vi "CRYAPI MANAGER.vi"(6 "cSpliterPos":T2(array[cluster]), 8 "tFrame":T3, 9 "sData":string, 10 "nData":i32, 11 "sAction":string) -> (1 "nData_Out":i32, 3 "tFrame_Out":T3)   [LabVIEW 2013]
uses:
  <vilib>/Utility/miscctls.llb/LVRectTypeDef.ctl
  CRYMain Sub Window Global.vi
panel:
  in  "nDocID":i32
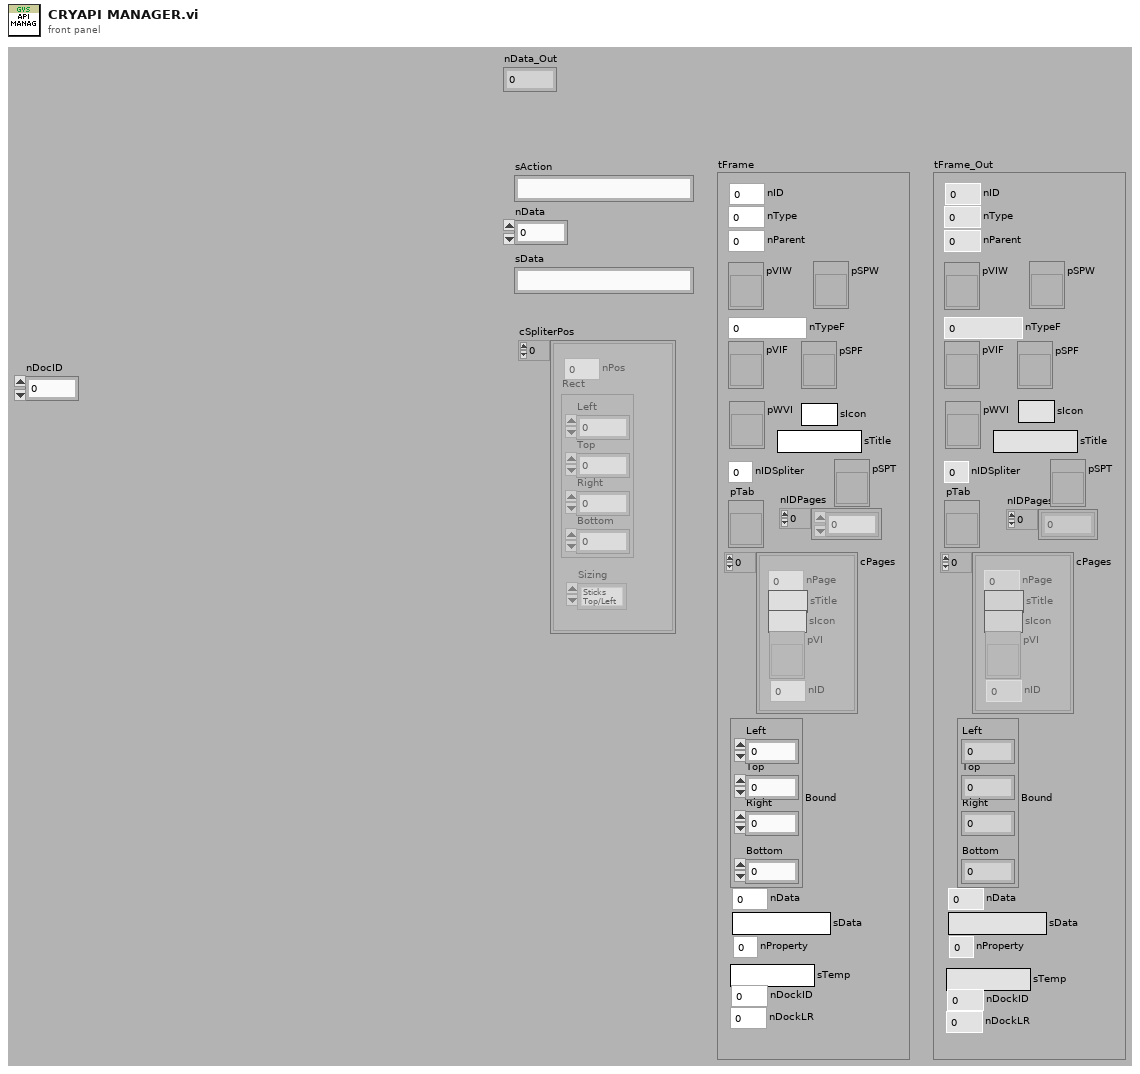
[diagram p1: front panel]
types:
  T1 = typedef "LVRectTypeDef.ctl" = cluster{"Left":i16, "Top":i16, "Right":i16, "Bottom":i16}
  T2 = cluster{"nPos":i32, "Rect":T1, "Sizing":enum16{"Sticks Top/Left", "Sticks Bottom/Right", "Proportional"}}[]
  T3 = cluster{"nType":i32, "nParent":i32, "pVIW":refnum<vi>, "pSPW":refnum<vi>, "nTypeF":i32, "pVIF":refnum<vi>, "pSPF":refnum<vi>, "nIDSpliter":i32, "nProperty":i32, "Bound":T1, "nID":i32, "nData":i32, "sData":string, "pWVI":refnum<vi>, "sTitle":string, "cPages":cluster{"nPage":i32, "sTitle":string, "sIcon":string, "pVI":refnum<vi>, "nID":i32}[], "pTab":refnum<vi>, "nIDPages":i32[], "pSPT":refnum<vi>, "sTemp":string, "nDockID":i32, "nDockLR":i32, "sIcon":string}
  T4 = enum16{"Sticks Top/Left", "Sticks Bottom/Right", "Proportional"}
  T5 = enum32{"Invalid", "Standard", "Closed", "Hidden", "Minimized", "Maximized"}
  T6 = enum32{"Invalid", "Default", "Floating", "Floating/Auto-Hide", "Modal"}
  T7 = cluster{"nPage":i32, "sTitle":string, "sIcon":string, "pVI":refnum<vi>, "nID":i32}[]
  T8 = cluster{"nID":i32[], "Frame":cluster{"nType":i32, "nParent":i32, "pVIW":refnum<vi>, "pSPW":refnum<vi>, "nTypeF":i32, "pVIF":refnum<vi>, "pSPF":refnum<vi>, "nIDSpliter":i32, "nProperty":i32, "Bound":T1, "nID":i32, "nData":i32, "sData":string, "pWVI":refnum<vi>, "sTitle":string, "cPages":cluster{"nPage":i32, "sTitle":string, "sIcon":string, "pVI":refnum<vi>, "nID":i32}[], "pTab":refnum<vi>, "nIDPages":i32[], "pSPT":refnum<vi>, "sTemp":string, "nDockID":i32, "nDockLR":i32, "sIcon":string}[]}
  T9 = cluster{"nType":i32, "nParent":i32, "pVIW":refnum<vi>, "pSPW":refnum<vi>, "nTypeF":i32, "pVIF":refnum<vi>, "pSPF":refnum<vi>, "nIDSpliter":i32, "nProperty":i32, "Bound":T1, "nID":i32, "nData":i32, "sData":string, "pWVI":refnum<vi>, "sTitle":string, "cPages":cluster{"nPage":i32, "sTitle":string, "sIcon":string, "pVI":refnum<vi>, "nID":i32}[], "pTab":refnum<vi>, "nIDPages":i32[], "pSPT":refnum<vi>, "sTemp":string, "nDockID":i32, "nDockLR":i32, "sIcon":string}[]
  T10 = cluster{"nType":i32, "nTypeP":i32, "pVI":refnum<vi>, "pSpliter":refnum<vi>, "pSPL":refnum<vi>, "pVIL":refnum<vi>, "pSPR":refnum<vi>, "pVIR":refnum<vi>, "nIDTL":i32, "nIDL":i32, "nIDTR":i32, "nIDR":i32, "nID":i32, "nIDParent":i32, "nData":i32, "sData":string}
  T11 = cluster{"CLOSE_HIDE":i32, "CLOSE_CLOSE":i32, "DOCK_ENABLE":i32, "DOCK_DISABLE":i32, "FOCUS_SHOW":i32, "FOCUS_HIDE":i32}
  T12 = cluster{"pSP":refnum<vi>, "pVI":refnum<vi>, "nIDT":i32, "nID":i32, "nLR":i32}
  T13 = typedef "LVBoundsTypeDef.ctl" = cluster{"Width":u32, "Height":u32}
  T14 = cluster{"nID":i32, "sTiltle":string, "pVI":refnum<vi>, "pSP":refnum<vi>, "pTab":refnum<vi>, "pSPT":refnum<vi>, "nWinType":i32, "sIcon":string}
  T15 = cluster{"nID":i32[], "Spliter":cluster{"nType":i32, "nTypeP":i32, "pVI":refnum<vi>, "pSpliter":refnum<vi>, "pSPL":refnum<vi>, "pVIL":refnum<vi>, "pSPR":refnum<vi>, "pVIR":refnum<vi>, "nIDTL":i32, "nIDL":i32, "nIDTR":i32, "nIDR":i32, "nID":i32, "nIDParent":i32, "nData":i32, "sData":string}[]}
  T16 = cluster{"nType":i32, "nTypeP":i32, "pVI":refnum<vi>, "pSpliter":refnum<vi>, "pSPL":refnum<vi>, "pVIL":refnum<vi>, "pSPR":refnum<vi>, "pVIR":refnum<vi>, "nIDTL":i32, "nIDL":i32, "nIDTR":i32, "nIDR":i32, "nID":i32, "nIDParent":i32, "nData":i32, "sData":string}[]
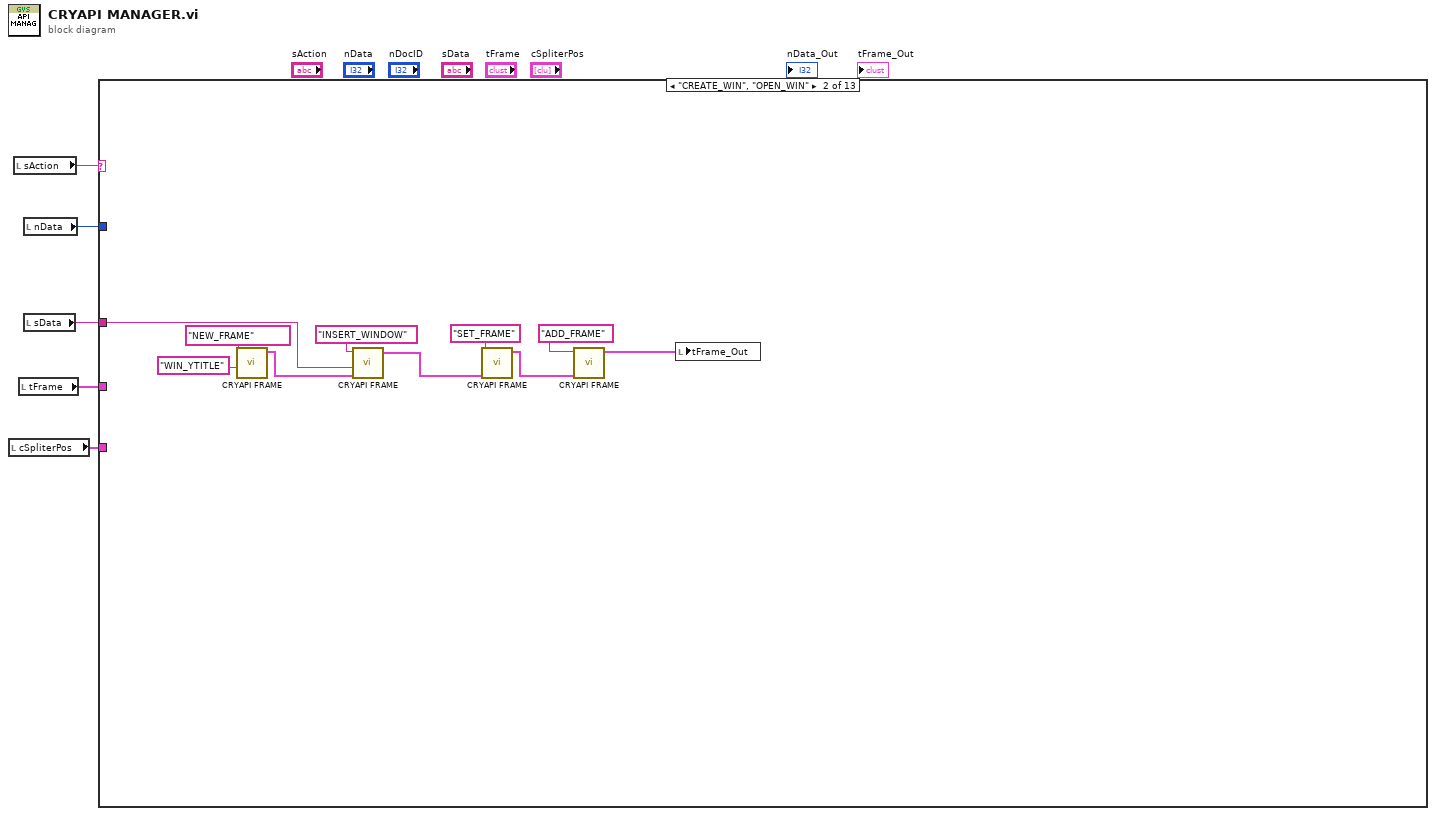
[diagram p0: block diagram]
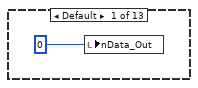
[diagram p2: hidden frame]
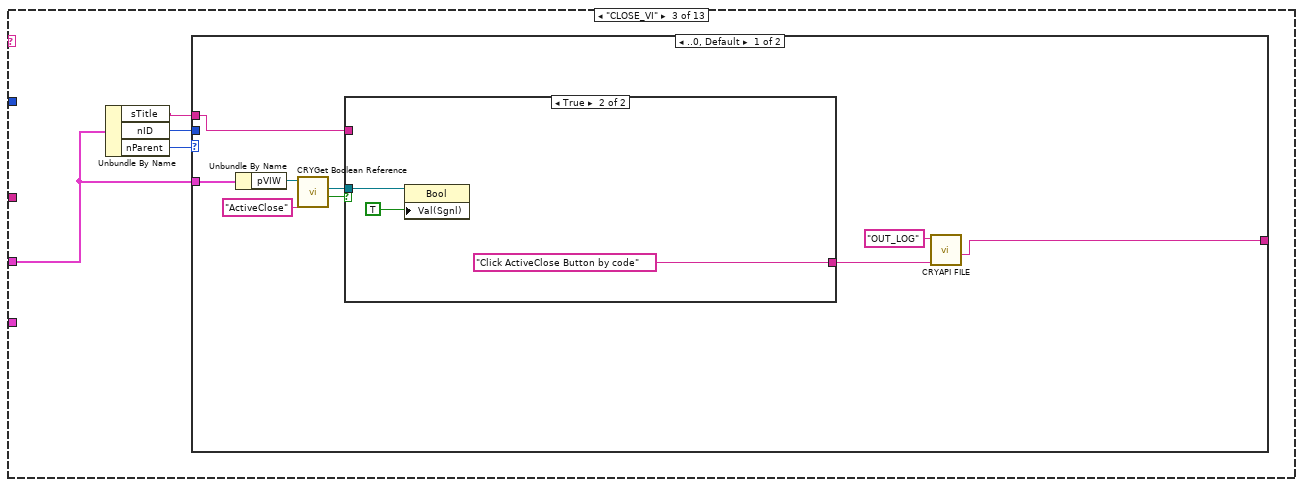
[diagram p3: hidden frame]
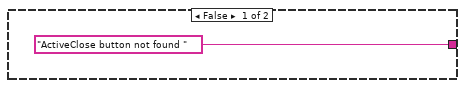
[diagram p4: hidden frame]
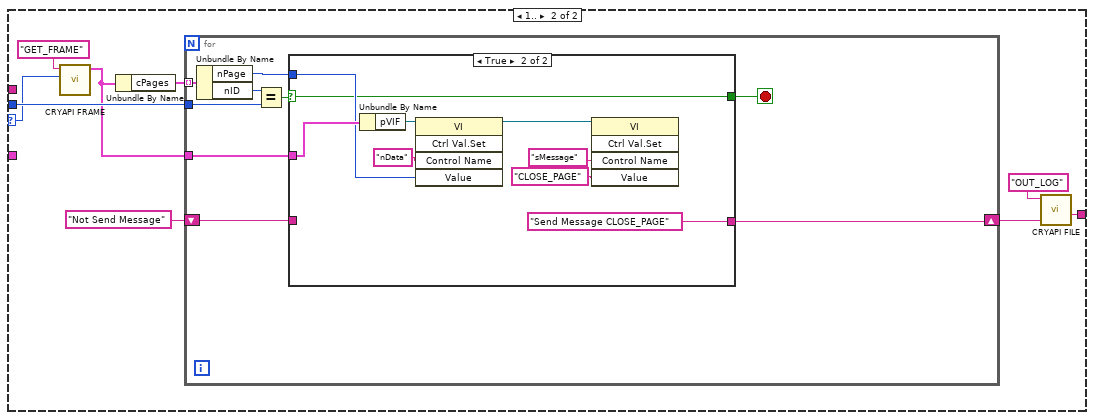
[diagram p5: hidden frame]
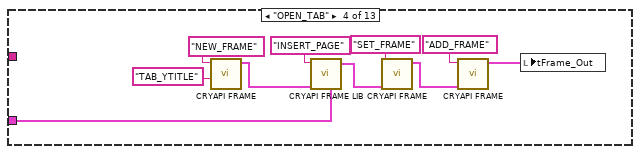
[diagram p7: hidden frame]
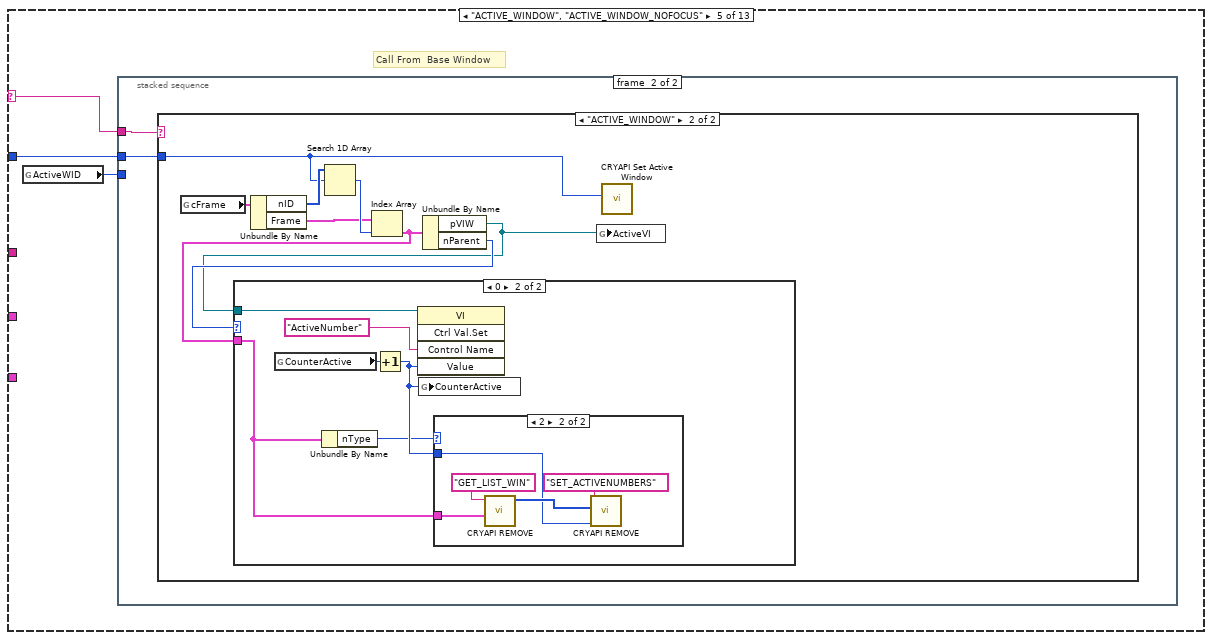
[diagram p8: hidden frame]
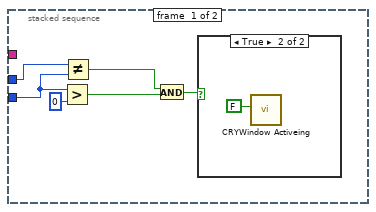
[diagram p9: hidden frame]
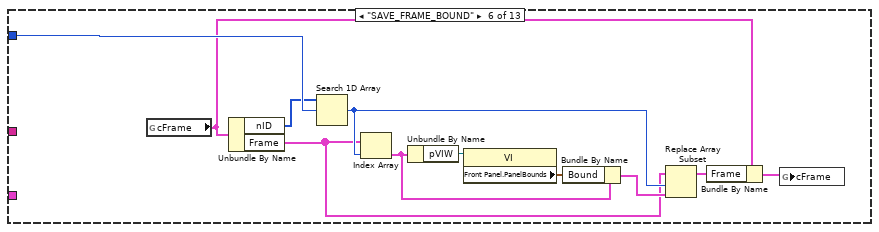
[diagram p14: hidden frame]
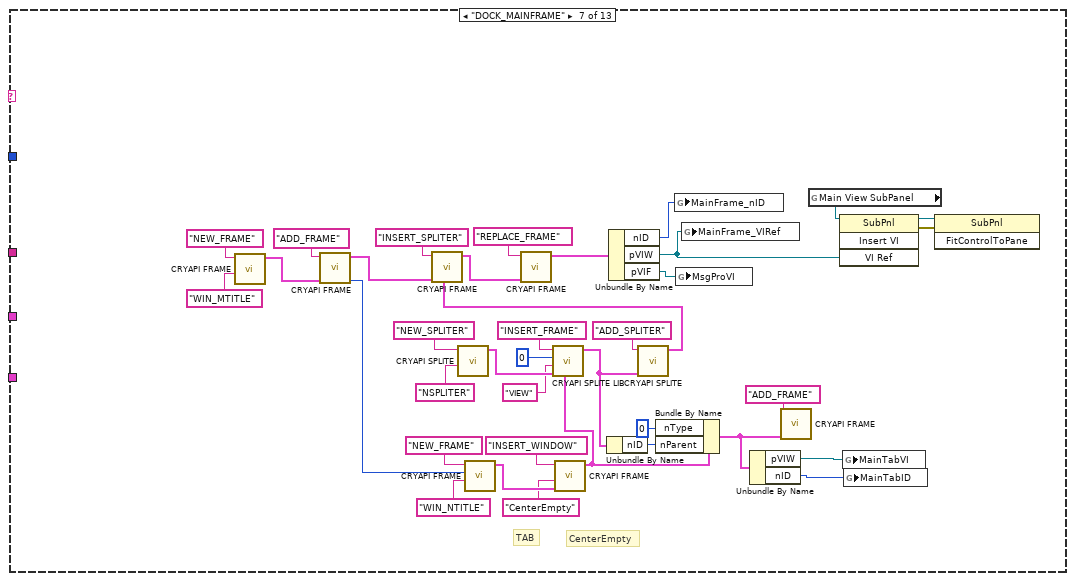
[diagram p15: hidden frame]
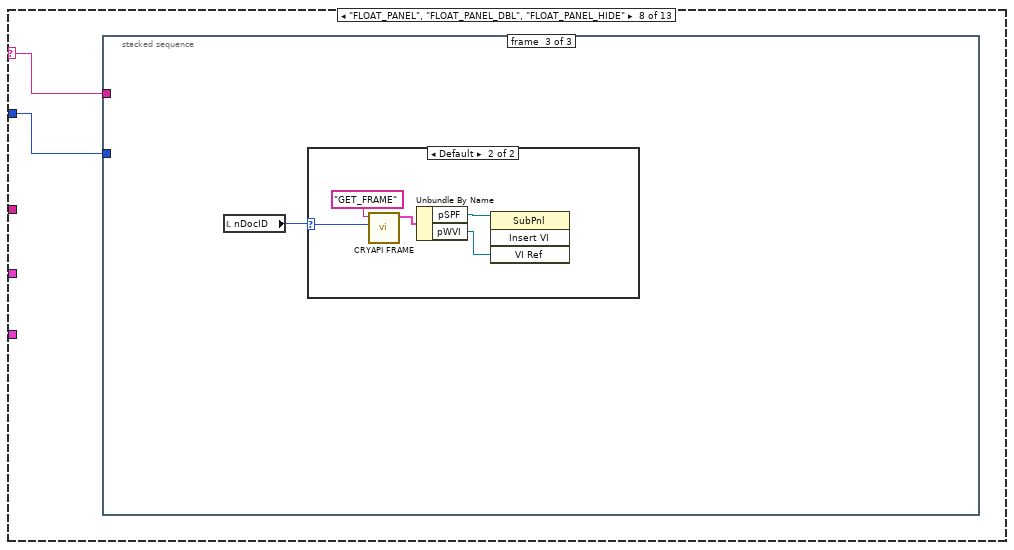
[diagram p16: hidden frame]
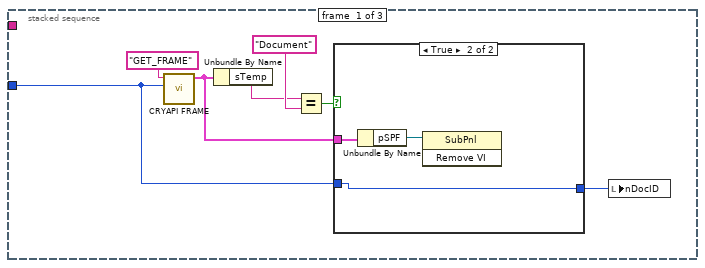
[diagram p17: hidden frame]
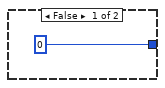
[diagram p18: hidden frame]
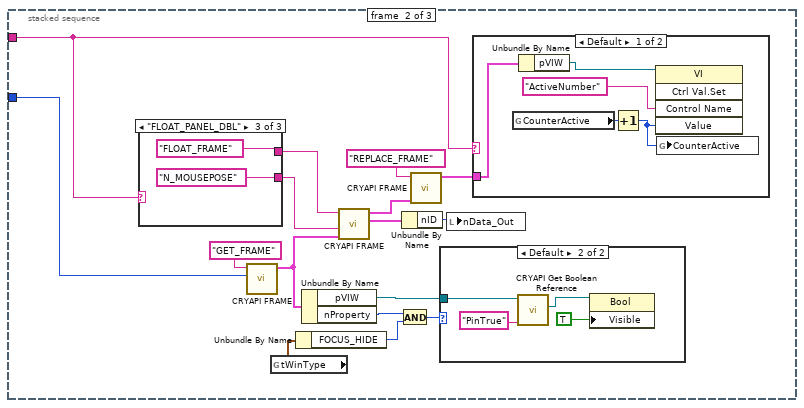
[diagram p19: hidden frame]
diagram:
  n1 = local read "cSpliterPos"() -> (w1:T2)
  n2 = local read "sAction"() -> (w5:string)
  n3 = local read "tFrame"() -> (w2:T3)
  n4 = local read "nData"() -> (w4:i32)
  n5 = local read "sData"() -> (w3:string)
  n6 = case shown="\"CREATE_WIN\", \"OPEN_WIN\"" w5 {
    selector: w5 -> [_ _ _ _ w74 _ _ w152 _ _ _ _ _]
    tunnel: w4 -> [_ _ _ _ w73 w113 _ w153 w204 w484 w591 w673 _]
    tunnel: w3 -> [_ w8 _ _ _ _ _ _ _ _ _ _ _]
    tunnel: w2 -> [_ _ w17 w65 _ _ _ _ w205 _ _ _ _]
    tunnel: w1 -> [_ _ _ _ _ _ _ _ _ _ w592 _ _]
    frame Default {
      n7 = local write "nData_Out"(0 ("nData_Out")) -> ()
    }
    frame "CREATE_WIN", "OPEN_WIN" {
      n8 = call "CRYAPI FRAME.vi"("sData"="WIN_YTITLE", "sAction"="NEW_FRAME") -> ("tFrame_Out"=w13:T3)  [unwired: 4 in, 5 out]
      n9 = call "CRYAPI FRAME.vi"("tFrame"=w13, "sData"=w8, "sAction"="INSERT_WINDOW" ("string")) -> ("tFrame_Out"=w12:T3)  [unwired: 3 in, 5 out]
      n10 = call "CRYAPI FRAME.vi"("tFrame"=w12, "sAction"="SET_FRAME" ("string")) -> ("tFrame_Out"=w9:T3)  [unwired: 4 in, 5 out]
      n11 = call "CRYAPI FRAME.vi"("tFrame"=w9, "sAction"="ADD_FRAME" ("string")) -> ("tFrame_Out"=w7:T3)  [unwired: 4 in, 5 out]
      n12 = local write "tFrame_Out"(w7) -> ()
    }
    frame "CLOSE_VI" {
      n13 = Unbundle By Name(w17) -> ("sTitle"=w18:string, "nID"=w19:i32, "nParent"=w20:i32)
      n14 = case shown="..0, Default" w20 {
        selector: w20 -> [_ w40]
        tunnel: w17 -> [w29 _]
        tunnel: w19 -> [_ w42]
        tunnel: [w22 w34] -> _
        tunnel: w18 -> [w21 _]
        frame ..0, Default {
          n15 = Unbundle By Name(w29) -> ("pVIW"=w28:refnum<vi>)
          n16 = call "CRYGet Boolean Reference.vi"("Label Name"="ActiveClose", "VI Refnum"=w28) -> ("Exist?"=w26:bool, "Boolean Ref"=w25:refnum<vi>)  [unwired: 8 out]
          n17 = case shown="True" w26 {
            tunnel: w25 -> [_ w33]
            tunnel: w21 -> [_ _]
            tunnel: ["ActiveClose button not found " ("sData") "Click ActiveClose Button by code" ("sData")] -> w23
            frame False {
            }
            frame True {
              n18 = property class="Bool"(reference=w33, "Val(Sgnl)"=TRUE) -> ()  [unwired: 1 in, 2 out]
            }
          }
          n19 = call "CRYAPI FILE.vi"("sData"=w23, "sAction"="OUT_LOG") -> ("sData_Out"=w22:string)  [unwired: 8 in, 1 out]
        }
        frame 1.. {
          n20 = call "CRYAPI FRAME.vi"("nData"=w40, "sAction"="GET_FRAME") -> ("tFrame_Out"=w38:T3)  [unwired: 4 in, 5 out]
          n21 = Unbundle By Name(w38) -> ("cPages"=w39:T7)
          n22 = for {
            tunnel: w39 -> [w51] mode=indexing
            tunnel: w42 -> [w49]
            tunnel: w38 -> [w47]
            shift-right: [w43] -> w35
            shift-left: "Not Send Message" ("Control Name") -> [w44]
            stop <- w45 stop-if-true
            n23 = Unbundle By Name(w51) -> ("nPage"=w46:i32, "nID"=w50:i32)
            n24 = Equal?(x=w50, y=w49) -> (x = y?=w48:bool)
            n25 = case shown="True" w48 {
              selector: w48 -> [w53 w55]
              tunnel: w47 -> [_ w57]
              tunnel: w46 -> [_ w56]
              tunnel: [w53 w55] -> w45
              tunnel: w44 -> [w52 _]
              tunnel: [w52 "Send Message CLOSE_PAGE" ("Control Name")] -> w43
              frame False {
              }
              frame True {
                n26 = Unbundle By Name(w57) -> ("pVIF"=w62:refnum<vi>)
                n27 = invoke class="VI" method="Ctrl Val.Set"(reference=w62, "Control Name"="nData", "Value"=w56) -> (reference out=w59:refnum<vi>)  [unwired: 2 in, 4 out]
                n28 = invoke class="VI" method="Ctrl Val.Set"(reference=w59, "Control Name"="sMessage", "Value"="CLOSE_PAGE" ("Control Name")) -> ()  [unwired: 2 in, 5 out]
              }
            }
          }
          n29 = call "CRYAPI FILE.vi"("sData"=w35, "sAction"="OUT_LOG") -> ("sData_Out"=w34:string)  [unwired: 8 in, 1 out]
        }
      }
    }
    frame "OPEN_TAB" {
      n30 = call "CRYAPI FRAME.vi"("sData"="TAB_YTITLE", "sAction"="NEW_FRAME") -> ("tFrame_Out"=w69:T3)  [unwired: 4 in, 5 out]
      n31 = call "CRYAPI FRAME LIB.vi"("tFrame_In"=w65, "tFrame"=w69, "sAction"="INSERT_PAGE" ("string")) -> ("tFrame_Out"=w64:T3)  [unwired: 3 in, 5 out]
      n32 = call "CRYAPI FRAME.vi"("tFrame"=w64, "sAction"="SET_FRAME" ("string")) -> ("tFrame_Out"=w66:T3)  [unwired: 4 in, 5 out]
      n33 = call "CRYAPI FRAME.vi"("tFrame"=w66, "sAction"="ADD_FRAME" ("string")) -> ("tFrame_Out"=w63:T3)  [unwired: 4 in, 5 out]
      n34 = local write "tFrame_Out"(w63) -> ()
    }
    frame "ACTIVE_WINDOW", "ACTIVE_WINDOW_NOFOCUS" {
      # "Call From  Base Window"
      n35 = global read "CRYMain Sub Window Global.vi" "ActiveWID"() -> (w75:i32)
      n36 = stacked-sequence {
        tunnel: w74 -> [_ w84]
        tunnel: w73 -> [w79 w83]
        tunnel: w75 -> [w80 _]
        frame #0 {
          n37 = Greater?(x=w80, y=0) -> (0:w76:bool)
          n38 = Not Equal?(x=w79, y=w80) -> (x != y?=w77:bool)
          n39 = And(x=w77, y=w76) -> (x .and. y?=w78:bool)
          n40 = case shown="True" w78 {
            frame False {
            }
            frame True {
              n41 = call "CRYWindow Activeing.vi"("ActiveTF"=FALSE) -> ()  [unwired: 11 in]
            }
          }
        }
        frame #1 {
          n42 = case shown="\"ACTIVE_WINDOW\"" w84 {
            tunnel: w83 -> [_ w85]
            frame "False", Default {
            }
            frame "ACTIVE_WINDOW" {
              n43 = global read "CRYMain Sub Window Global.vi" "cFrame"() -> (w91:T8)
              n44 = Unbundle By Name(w91) -> ("nID"=w90:i32[], "Frame"=w89:T9)
              n45 = Search 1D Array(1D array=w90, element=w85) -> (index of element=w92:i32)  [unwired: 1 out]
              n46 = Index Array(array=w89, index=w92) -> (element=w86:T3)
              n47 = Unbundle By Name(w86) -> ("pVIW"=w87:refnum<vi>, "nParent"=w88:i32)
              n48 = case shown="0" w88 {
                tunnel: w87 -> [_ w96]
                tunnel: w86 -> [_ w93]
                frame Default {
                }
                frame 0 {
                  n49 = global read "CRYMain Sub Window Global.vi" "CounterActive"() -> (w97:i32)
                  n50 = Unbundle By Name(w93) -> ("nType"=w94:i32)
                  n51 = Increment(x=w97) -> (x+1=w95:i32)
                  n52 = invoke class="VI" method="Ctrl Val.Set"(reference=w96, "Control Name"="ActiveNumber", "Value"=w95) -> ()  [unwired: 2 in, 5 out]
                  n53 = global write "CRYMain Sub Window Global.vi" "CounterActive"(w95) -> ()
                  n54 = case shown="2" w94 {
                    tunnel: w93 -> [_ w100]
                    tunnel: w95 -> [_ w99]
                    frame Default {
                    }
                    frame 2 {
                      n55 = call "CRYAPI REMOVE.vi"("tFrame"=w100, "sAction"="GET_LIST_WIN") -> ("List_ID_Out"=w101:i32[])  [unwired: 3 in, 6 out]
                      n56 = call "CRYAPI REMOVE.vi"("nData"=w99, "List_ID"=w101, "sAction"="SET_ACTIVENUMBERS") -> ()  [unwired: 2 in, 7 out]
                    }
                  }
                }
              }
              n57 = global write "CRYMain Sub Window Global.vi" "ActiveVI"(w87) -> ()
              n58 = call "CRYAPI Set Active Window.vi"("nData"=w85) -> ()  [unwired: 11 in]
            }
          }
        }
      }
    }
    frame "SAVE_FRAME_BOUND" {
      n59 = global read "CRYMain Sub Window Global.vi" "cFrame"() -> (w112:T8)
      n60 = Unbundle By Name(w112) -> ("nID"=w111:i32[], "Frame"=w105:T9)
      n61 = Search 1D Array(1D array=w111, element=w113) -> (index of element=w107:i32)  [unwired: 1 out]
      n62 = Index Array(array=w105, index=w107) -> (element=w109:T3)
      n63 = Unbundle By Name(w109) -> ("pVIW"=w110:refnum<vi>)
      n64 = property class="VI"(reference=w110) -> ("Front Panel.PanelBounds"=w108:T1)  [unwired: 1 in, 2 out]
      n65 = Bundle By Name(cluster=w109, "Bound"=w108) -> (w106:T3)
      n66 = Replace Array Subset(array=w105, new element=w106, index=w107) -> (w104:T9)
      n67 = Bundle By Name(cluster=w112, "Frame"=w104) -> (w114:T8)
      n68 = global write "CRYMain Sub Window Global.vi" "cFrame"(w114) -> ()
    }
    frame "DOCK_MAINFRAME" {
      # "CenterEmpty"
      # "TAB"
      n69 = call "CRYAPI FRAME.vi"("sData"="WIN_MTITLE", "sAction"="NEW_FRAME") -> ("tFrame_Out"=w148:T3)  [unwired: 4 in, 5 out]
      n70 = call "CRYAPI FRAME.vi"("tFrame"=w148, "sAction"="ADD_FRAME") -> ("nData_Out"=w121:i32, "tFrame_Out"=w130:T3)  [unwired: 4 in, 4 out]
      n71 = call "CRYAPI SPLITE.vi"("sData"="NSPLITER", "sAction"="NEW_SPLITER") -> ("tSpliter_Out"=w135:T10)  [unwired: 4 in, 5 out]
      n72 = call "CRYAPI FRAME.vi"("sData"="WIN_NTITLE", "nData"=w121, "sAction"="NEW_FRAME") -> ("tFrame_Out"=w139:T3)  [unwired: 3 in, 5 out]
      n73 = call "CRYAPI FRAME.vi"("tFrame"=w139, "sData"="CenterEmpty", "sAction"="INSERT_WINDOW" ("string")) -> ("tFrame_Out"=w124:T3)  [unwired: 3 in, 5 out]
      n74 = call "CRYAPI SPLITE LIB.vi"("tFrame"=w124, "tSpliter"=w135, "sData"="VIEW", "nData"=0, "sAction"="INSERT_FRAME") -> ("tSpliter_Out"=w125:T10)  [unwired: 1 in, 5 out]
      n75 = Unbundle By Name(w125) -> ("nID"=w126:i32)
      n76 = call "CRYAPI SPLITE.vi"("tSpliter"=w125, "sAction"="ADD_SPLITER") -> ("tSpliter_Out"=w122:T10)  [unwired: 4 in, 5 out]
      n77 = call "CRYAPI FRAME.vi"("tSpliter"=w122, "tFrame"=w130, "sAction"="INSERT_SPLITER") -> ("tFrame_Out"=w129:T3)  [unwired: 3 in, 5 out]
      n78 = call "CRYAPI FRAME.vi"("tFrame"=w129, "sAction"="REPLACE_FRAME") -> ("tFrame_Out"=w127:T3)  [unwired: 4 in, 5 out]
      n79 = Unbundle By Name(w127) -> ("nID"=w145:i32, "pVIW"=w115:refnum<vi>, "pVIF"=w119:refnum<vi>)
      n80 = Bundle By Name(cluster=w124, "nType"=0, "nParent"=w126) -> (w118:T3)
      n81 = global write "CRYMain Sub Window Global.vi" "MainFrame_nID"(w145) -> ()
      n82 = global write "CRYMain Sub Window Global.vi" "MsgProVI"(w119) -> ()
      n83 = global write "CRYMain Sub Window Global.vi" "MainFrame_VIRef"(w115) -> ()
      n84 = Unbundle By Name(w118) -> ("pVIW"=w117:refnum<vi>, "nID"=w116:i32)
      n85 = call "CRYAPI FRAME.vi"("tFrame"=w118, "sAction"="ADD_FRAME" ("string")) -> ()  [unwired: 4 in, 6 out]
      n86 = global read "CRYMain Sub Window Global.vi" "Main View SubPanel"() -> (w146:refnum<vi>)
      n87 = invoke class="SubPnl" method="Insert VI"(reference=w146, "VI Ref"=w115) -> (reference out=w147:refnum<vi>, error out=w144:errorcluster)  [unwired: 2 in, 2 out]
      n88 = global write "CRYMain Sub Window Global.vi" "MainTabVI"(w117) -> ()
      n89 = global write "CRYMain Sub Window Global.vi" "MainTabID"(w116) -> ()
      n90 = invoke class="SubPnl" method="FitControlToPane"(reference=w147, error in=w144) -> ()  [unwired: 1 in, 3 out]
    }
    frame "FLOAT_PANEL", "FLOAT_PANEL_DBL", "FLOAT_PANEL_HIDE" {
      n91 = stacked-sequence {
        tunnel: w153 -> [w154 w175 _]
        tunnel: w152 -> [_ w171 _]
        frame #0 {
          n92 = call "CRYAPI FRAME.vi"("nData"=w154, "sAction"="GET_FRAME") -> ("tFrame_Out"=w159:T3)  [unwired: 4 in, 5 out]
          n93 = Unbundle By Name(w159) -> ("sTemp"=w156:string)
          n94 = Equal?(x=w156, y="Document" ("Window Type")) -> (x = y?=w158:bool)
          n95 = case shown="True" w158 {
            tunnel: w159 -> [_ w164]
            tunnel: w154 -> [_ w162]
            tunnel: [0 ("nData") w162] -> w160
            frame False {
            }
            frame True {
              n96 = Unbundle By Name(w164) -> ("pSPF"=w163:refnum<vi>)
              n97 = invoke class="SubPnl" method="Remove VI"(reference=w163) -> ()  [unwired: 2 in, 3 out]
            }
          }
          n98 = local write "nDocID"(w160) -> ()
        }
        frame #1 {
          n99 = case shown="\"FLOAT_PANEL_DBL\"" w171 {
            tunnel: ["FLOAT_FRAME" ("sAction") "FLOAT_FRAME_HIDE" ("sAction") "FLOAT_FRAME" ("sAction")] -> w178
            tunnel: ["MOUSEPOSE" ("sData") "MOUSEPOSE" ("sData") "N_MOUSEPOSE" ("sData")] -> w177
            frame Default {
            }
            frame "FLOAT_PANEL_HIDE" {
            }
            frame "FLOAT_PANEL_DBL" {
            }
          }
          n100 = call "CRYAPI FRAME.vi"("nData"=w175, "sAction"="GET_FRAME") -> ("tFrame_Out"=w165:T3)  [unwired: 4 in, 5 out]
          n101 = global read "CRYMain Sub Window Global.vi" "tWinType"() -> (w166:T11)
          n102 = Unbundle By Name(w166) -> ("FOCUS_HIDE"=w168:i32)
          n103 = Unbundle By Name(w165) -> ("pVIW"=w170:refnum<vi>, "nProperty"=w167:i32)
          n104 = call "CRYAPI FRAME.vi"("tFrame"=w165, "sData"=w177, "sAction"=w178) -> ("tSpliter_Out"=w176:T10, "tFrame_Out"=w174:T3)  [unwired: 3 in, 4 out]
          n105 = And(x=w167, y=w168) -> (x .and. y?=w169:i32)
          n106 = Unbundle By Name(w176) -> ("nID"=w180:i32)
          n107 = call "CRYAPI FRAME.vi"("tFrame"=w174, "sAction"="REPLACE_FRAME") -> ("tFrame_Out"=w172:T3)  [unwired: 4 in, 5 out]
          n108 = case shown="Default" w169 {
            tunnel: w170 -> [_ w182]
            frame 0 {
            }
            frame Default {
              n109 = call "CRYAPI Get Boolean Reference.vi"("Label Name"="PinTrue", "VI Refnum"=w182) -> ("Boolean Ref"=w183:refnum<vi>)  [unwired: 9 out]
              n110 = property class="Bool"(reference=w183, "Visible"=TRUE) -> ()  [unwired: 1 in, 2 out]
            }
          }
          n111 = local write "nData_Out"(w180) -> ()
          n112 = case shown="Default" w171 {
            tunnel: w172 -> [w186 _]
            frame Default {
              n113 = global read "CRYMain Sub Window Global.vi" "CounterActive"() -> (w188:i32)
              n114 = Unbundle By Name(w186) -> ("pVIW"=w185:refnum<vi>)
              n115 = Increment(x=w188) -> (x+1=w189:i32)
              n116 = invoke class="VI" method="Ctrl Val.Set"(reference=w185, "Control Name"="ActiveNumber", "Value"=w189) -> ()  [unwired: 2 in, 5 out]
              n117 = global write "CRYMain Sub Window Global.vi" "CounterActive"(w189) -> ()
            }
            frame "FLOAT_PANEL_HIDE" {
            }
          }
        }
        frame #2 {
          n118 = local read "nDocID"() -> (w196:i32)
          n119 = case shown="Default" w196 {
            selector: w196 -> [_ w200]
            frame 0 {
            }
            frame Default {
              n120 = call "CRYAPI FRAME.vi"("nData"=w200, "sAction"="GET_FRAME") -> ("tFrame_Out"=w199:T3)  [unwired: 4 in, 5 out]
              n121 = Unbundle By Name(w199) -> ("pSPF"=w198:refnum<vi>, "pWVI"=w197:refnum<vi>)
              n122 = invoke class="SubPnl" method="Insert VI"(reference=w198, "VI Ref"=w197) -> ()  [unwired: 2 in, 4 out]
            }
          }
        }
      }
    }
    frame "FLOAT_FRAME" {
      n123 = call "CRYAPI SPLITE LIB.vi"("nData"=w204, "sAction"="CHECK_ROOT") -> ("nData_Out"=w202:i32)  [unwired: 4 in, 5 out]
      n124 = case shown="0, Default" w202 {
        tunnel: w205 -> [w210 w362]
        tunnel: w204 -> [w219 w363]
        frame 0, Default {
          n125 = global read "CRYMain Sub Window Global.vi" "MainFrame_nID"() -> (w220:i32)
          n126 = call "CRYAPI SPLITE.vi"("nData"=w219, "sAction"="GET_SPLITER") -> ("tSpliter_Out"=w209:T10)  [unwired: 4 in, 5 out]
          n127 = call "CRYAPI FRAME.vi"("nData"=w220, "sAction"="GET_FRAME") -> ("tFrame_Out"=w214:T3)  [unwired: 4 in, 5 out]
          n128 = Unbundle By Name(w214) -> ("nIDSpliter"=w217:i32)
          n129 = call "CRYAPI REMOVE.vi"("tFrame"=w214, "sAction"="GET_LIST_ID") -> ("List_ID_Out"=w218:i32[])  [unwired: 3 in, 6 out]
          n130 = call "CRYAPI SPLITE.vi"("tFrame"=w210, "tSpliter"=w209, "sAction"="GET_FRAME_XLR") -> ("tLR_Out"=w211:T12)  [unwired: 3 in, 5 out]
          n131 = call "CRYAPI SPLITE.vi"("tFrame"=w210, "tSpliter"=w209, "sAction"="GET_FRAME_LR") -> ("tLR_Out"=w208:T12)  [unwired: 3 in, 5 out]
          n132 = local write "tFrame_Out"(w210) -> ()
          n133 = Unbundle By Name(w208) -> ("pSP"=w207:refnum<vi>)
          n134 = Insert Into Array(array=w218, index=0, new element=w217) -> (w215:i32[])
          n135 = Equal?(x=w217, y=w219) -> (x = y?=w206:bool)
          n136 = case shown="False" w206 {
            tunnel: w211 -> [w232 w256]
            tunnel: w209 -> [w231 w255]
            tunnel: w215 -> [_ w260]
            tunnel: w219 -> [_ w257]
            tunnel: w214 -> [w230 _]
            tunnel: w207 -> [_ w254]
            frame True {
              n137 = Unbundle By Name(w232) -> ("nID"=w227:i32, "pVI"=w236:refnum<vi>, "pSP"=w233:refnum<vi>)
              n138 = Unbundle By Name(w230) -> ("pSPF"=w229:refnum<vi>)
              n139 = invoke class="SubPnl" method="Remove VI"(reference=w229) -> (reference out=w234:refnum<vi>)  [unwired: 2 in, 2 out]
              n140 = invoke class="SubPnl" method="Remove VI"(reference=w233) -> (reference out=w235:refnum<vi>)  [unwired: 2 in, 2 out]
              n141 = call "CRYAPI SPLITE.vi"("nData"=w227, "sAction"="GET_SPLITER") -> ("tSpliter_Out"=w226:T10)  [unwired: 4 in, 5 out]
              n142 = stacked-sequence {
                tunnel: w234 -> [w252]
                tunnel: w235 -> [_]
                tunnel: w236 -> [w251]
                tunnel: w230 -> [w246]
                tunnel: w227 -> [w248]
                tunnel: w231 -> [w243]
                tunnel: [w243] -> w237
                tunnel: [w247] -> w240
                tunnel: w226 -> [w242]
                tunnel: [w241] -> w224
                frame #0 {
                  n143 = Unbundle By Name(w246) -> ("nID"=w245:i32)
                  n144 = invoke class="SubPnl" method="Insert VI"(reference=w252, "VI Ref"=w251) -> (reference out=w250:refnum<vi>, error out=w249:errorcluster)  [unwired: 2 in, 2 out]
                  n145 = Bundle By Name(cluster=w246, "nIDSpliter"=w248) -> (w247:T3)
                  n146 = Bundle By Name(cluster=w242, "nIDParent"=w245, "nTypeP"=0) -> (w241:T10)
                  n147 = invoke class="SubPnl" method="FitControlToPane"(reference=w250, error in=w249) -> ()  [unwired: 1 in, 3 out]
                }
              }
              n148 = call "CRYAPI FRAME.vi"("tFrame"=w240, "sAction"="REPLACE_FRAME") -> ()  [unwired: 4 in, 6 out]
              n149 = call "CRYAPI SPLITE.vi"("tSpliter"=w237, "sAction"="REMOVE_SPLITER") -> ()  [unwired: 4 in, 6 out]
              n150 = call "CRYAPI SPLITE.vi"("tSpliter"=w224, "sAction"="REPLACE_SPLITER") -> ()  [unwired: 4 in, 6 out]
            }
            frame False {
              n151 = property class="SubPnl"(reference=w254) -> ("Bounds"=w253:T13)  [unwired: 1 in, 2 out]
              n152 = call "CRYAPI REMOVE.vi"("nData"=w257, "List_ID"=w260, "sAction"="FIND_SPLITER") -> ("nData_Out"=w259:i32, "tSpliter_Out"=w258:T10)  [unwired: 2 in, 5 out]
              n153 = case shown="Default" w259 {
                tunnel: w258 -> [_ w271]
                tunnel: w257 -> [_ w281]
                tunnel: w256 -> [_ w278]
                tunnel: w255 -> [_ w280]
                tunnel: w253 -> [_ w273]
                frame -1 {
                  n154 = local write "nData_Out"(0 ("nData_Out")) -> ()
                }
                frame Default {
                  n155 = Unbundle By Name(w271) -> ("nType"=w267:i32, "pSpliter"=w270:refnum<vi>)
                  n156 = Unbundle By Name(w271) -> ("nType"=w274:i32)
                  n157 = case shown="0, 1, Default" w274 {
                    tunnel: w273 -> [w307 w309]
                    tunnel: [w306 w308] -> w272
                    frame 0, 1, Default {
                      n158 = Unbundle By Name(w307) -> ("Width"=w306:u32)
                    }
                    frame 2 {
                      n159 = Unbundle By Name(w309) -> ("Height"=w308:u32)
                    }
                  }
                  n160 = call "CRYAPI SPLITE.vi"("tSpliter"=w271, "nData"=w281, "sAction"="GET_ID_LR") -> ("nData_Out"=w283:i32)  [unwired: 3 in, 5 out]
                  n161 = case shown="1" w283 {
                    tunnel: w278 -> [w330 w343 w354]
                    tunnel: w271 -> [w329 w342 w353]
                    tunnel: [w335 w348 w359] -> w287
                    tunnel: [w334 w347 w358] -> w285
                    tunnel: [w333 w346 w357] -> w284
                    tunnel: w280 -> [w331 w344 w355]
                    tunnel: [w331 w344 w355] -> w289
                    tunnel: [w330 w343 w354] -> w276
                    tunnel: [w329 w342 w353] -> w275
                    tunnel: w272 -> [w328 w341 w352]
                    tunnel: [w328 w340 w352] -> w269
                    tunnel: [T4."Sticks Top/Left" ("Sizing") T4."Sticks Top/Left" ("Sizing") T4."Sticks Bottom/Right" ("Sizing")] -> w268
                    frame 0, Default {
                      n162 = Unbundle By Name(w330) -> ("pVI"=w334:refnum<vi>, "nIDT"=w337:i32, "nID"=w336:i32, "pSP"=w332:refnum<vi>)
                      n163 = invoke class="SubPnl" method="Remove VI"(reference=w332) -> ()  [unwired: 2 in, 3 out]
                      n164 = Unbundle By Name(w329) -> ("pSPL"=w333:refnum<vi>)
                      n165 = Bundle By Name(cluster=w329, "pVIL"=w334, "nIDTL"=w337, "nIDL"=w336) -> (w335:T10)
                    }
                    frame 1 {
                      n166 = Unbundle By Name(w343) -> ("pVI"=w347:refnum<vi>, "nIDT"=w350:i32, "nID"=w349:i32, "pSP"=w345:refnum<vi>)
                      n167 = Multiply(x=-1, y=w341) -> (x*y=w340:u32)
                      n168 = invoke class="SubPnl" method="Remove VI"(reference=w345) -> ()  [unwired: 2 in, 3 out]
                      n169 = Unbundle By Name(w342) -> ("pSPL"=w346:refnum<vi>)
                      n170 = Bundle By Name(cluster=w342, "pVIL"=w347, "nIDTL"=w350, "nIDL"=w349) -> (w348:T10)
                    }
                    frame 2 {
                      n171 = Unbundle By Name(w354) -> ("pVI"=w358:refnum<vi>, "nIDT"=w361:i32, "nID"=w360:i32, "pSP"=w356:refnum<vi>)
                      n172 = invoke class="SubPnl" method="Remove VI"(reference=w356) -> ()  [unwired: 2 in, 3 out]
                      n173 = Unbundle By Name(w353) -> ("pSPR"=w357:refnum<vi>)
                      n174 = Bundle By Name(cluster=w353, "pVIR"=w358, "nIDTR"=w361, "nIDR"=w360) -> (w359:T10)
                    }
                  }
                  n175 = case shown="1, 2" w267 {
                    tunnel: w270 -> [_ w303]
                    tunnel: w269 -> [_ w301]
                    tunnel: w268 -> [_ w296]
                    tunnel: [_ w296] -> w263
                    frame 0, Default {
                    }
                    frame 1, 2 {
                      n176 = property class="Splitter"(reference=w303) -> (reference out=w300:refnum<vi>, "Position"=w302:i32)  [unwired: 1 in, 1 out]
                      n177 = Add(x=w301, y=w302) -> (x+y=w299:u32)
                      n178 = property class="Splitter"(reference=w300, "Position"=w299) -> (reference out=w298:refnum<vi>, error out=w297:errorcluster)  [unwired: 1 in]
                      n179 = case shown="No Error" w297 {
                        tunnel: w298 -> [w305 _]
                        tunnel: w296 -> [w304 _]
                        frame No Error {
                          n180 = property class="Splitter"(reference=w305, "Sizing"=w304) -> ()  [unwired: 1 in, 2 out]
                        }
                        frame Error {
                        }
                      }
                    }
                  }
                  n181 = Unbundle By Name(w276) -> ("nID"=w277:i32, "nIDT"=w279:i32)
                  n182 = call "CRYAPI SPLITE.vi"("tSpliter"=w287, "sAction"="REPLACE_SPLITER") -> ("tSpliter_Out"=w266:T10)  [unwired: 4 in, 5 out]
                  n183 = case shown="0" w279 {
                    tunnel: w277 -> [w313 w323]
                    tunnel: w275 -> [w311 w321]
                    tunnel: [w310 w318] -> w264
                    frame 0 {
                      n184 = Unbundle By Name(w311) -> ("nID"=w317:i32)
                      n185 = call "CRYAPI FRAME.vi"("nData"=w313, "sAction"="GET_FRAME") -> ("tFrame_Out"=w312:T3)  [unwired: 4 in, 5 out]
                      n186 = Bundle By Name(cluster=w312, "nParent"=w317) -> (w315:T3)
                      n187 = call "CRYAPI FRAME.vi"("tFrame"=w315, "sAction"="REPLACE_FRAME") -> ("nData_Out"=w310:i32)  [unwired: 4 in, 5 out]
                    }
                    frame 1, Default {
                      n188 = Unbundle By Name(w321) -> ("nID"=w326:i32)
                      n189 = call "CRYAPI SPLITE.vi"("nData"=w323, "sAction"="GET_SPLITER") -> ("tSpliter_Out"=w322:T10)  [unwired: 4 in, 5 out]
                      n190 = Bundle By Name(cluster=w322, "nIDParent"=w326, "nTypeP"=1) -> (w320:T10)
                      n191 = call "CRYAPI SPLITE.vi"("tSpliter"=w320, "sAction"="REPLACE_SPLITER") -> ("nData_Out"=w318:i32)  [unwired: 4 in, 5 out]
                    }
                  }
                  n192 = call "CRYAPI SPLITE.vi"("tSpliter"=w289, "sAction"="REMOVE_SPLITER") -> ("tSpliter_Out"=w265:T10)  [unwired: 4 in, 5 out]
                  n193 = flat-sequence {
                    tunnel: w285 -> [w293]
                    tunnel: w284 -> [w290]
                    tunnel: w266 -> [_]
                    tunnel: w265 -> [_]
                    tunnel: w264 -> [_]
                    tunnel: w263 -> [_]
                    frame #0 {
                      n194 = invoke class="SubPnl" method="Remove VI"(reference=w290) -> (reference out=w291:refnum<vi>, error out=w292:errorcluster)  [unwired: 2 in, 1 out]
                      n195 = invoke class="SubPnl" method="Insert VI"(reference=w291, error in=w292, "VI Ref"=w293) -> (reference out=w294:refnum<vi>, error out=w295:errorcluster)  [unwired: 1 in, 2 out]
                      n196 = invoke class="SubPnl" method="FitControlToPane"(reference=w294, error in=w295) -> ()  [unwired: 1 in, 3 out]
                    }
                  }
                }
              }
            }
          }
        }
        frame 1 {
          n197 = call "CRYAPI SPLITE.vi"("nData"=w363, "sAction"="GET_SPLITER") -> ("tSpliter_Out"=w369:T10)  [unwired: 4 in, 5 out]
          n198 = call "CRYAPI SPLITE.vi"("tFrame"=w362, "tSpliter"=w369, "sAction"="GET_FRAME_XLR") -> ("tLR_Out"=w368:T12, "tSpliter_Out"=w366:T10)  [unwired: 3 in, 4 out]
          n199 = local write "tFrame_Out"(w362) -> ()
          n200 = Unbundle By Name(w366) -> ("sData"=w367:string)
          n201 = case shown="\"FRAME\", Default" w367 {
            tunnel: w368 -> [w392 w414 w439]
            tunnel: w369 -> [w391 w400 w435]
            tunnel: w362 -> [w390 _ _]
            frame "FRAME", Default {
              n202 = Unbundle By Name(w392) -> ("nID"=w385:i32)
              n203 = call "CRYAPI FRAME.vi"("nData"=w385, "sAction"="GET_FRAME") -> ("tFrame_Out"=w389:T3)  [unwired: 4 in, 5 out]
              n204 = Unbundle By Name(w390) -> ("pVIW"=w379:refnum<vi>)
              n205 = property class="VI"(reference=w379) -> ("FP.State"=w378:T5)  [unwired: 1 in, 2 out]
              n206 = call "CRYAPI FRAME.vi"("tFrame"=w389, "sData"="NO_MOUSEPOSE", "sAction"="FLOAT_FRAME") -> ("nData_Out"=w381:i32, "tFrame_Out"=w380:T3)  [unwired: 3 in, 4 out]
              n207 = Equal?(x=T5."Standard" ("Front Panel Window:State"), y=w378) -> (x = y?=w376:bool)
              n208 = case shown="True" w376 {
                tunnel: w381 -> [_ w393]
                tunnel: w390 -> [_ w394]
                frame False {
                }
                frame True {
                  n209 = stacked-sequence {
                    tunnel: w394 -> [w395]
                    tunnel: w393 -> [_]
                    frame #0 {
                      n210 = Unbundle By Name(w395) -> ("pVIW"=w398:refnum<vi>)
                      n211 = property class="VI"(reference=w398, "FP.Behavior"=T6."Floating" ("Front Panel Window:Behavior"), "FP.State"=T5."Standard" ("Front Panel Window:State")) -> ()  [unwired: 1 in, 2 out]
                    }
                  }
                }
              }
              n212 = Unbundle By Name(w391) -> ("nIDParent"=w373:i32)
              n213 = call "CRYAPI FRAME.vi"("tFrame"=w380, "sAction"="SET_DOCK") -> ("tFrame_Out"=w382:T3)  [unwired: 4 in, 5 out]
              n214 = call "CRYAPI FRAME.vi"("tFrame"=w380, "nData"=w373, "sAction"="GET_FRAME") -> ("tFrame_Out"=w372:T3)  [unwired: 3 in, 5 out]
              n215 = call "CRYAPI FRAME.vi"("tFrame"=w382, "sAction"="REPLACE_FRAME") -> ()  [unwired: 4 in, 6 out]
              n216 = call "CRYAPI FRAME.vi"("tFrame"=w372, "sAction"="REMOVE_FRAME") -> ("nData_Out"=w375:i32)  [unwired: 4 in, 5 out]
              n217 = call "CRYAPI SPLITE.vi"("tSpliter"=w391, "nData"=w375, "sAction"="REMOVE_SPLITER") -> ()  [unwired: 3 in, 6 out]
            }
            frame "ROOT" {
              n218 = Unbundle By Name(w400) -> ("nIDParent"=w416:i32)
              n219 = Unbundle By Name(w414) -> ("pSP"=w413:refnum<vi>, "pVI"=w412:refnum<vi>, "nID"=w410:i32)
              n220 = call "CRYAPI FRAME.vi"("nData"=w416, "sAction"="GET_FRAME") -> ("nData_Out"=w399:i32, "tFrame_Out"=w415:T3)  [unwired: 4 in, 4 out]
              n221 = invoke class="SubPnl" method="Remove VI"(reference=w413) -> (error out=w403:errorcluster)  [unwired: 2 in, 2 out]
              n222 = Bundle By Name(cluster=w415, "nIDSpliter"=w410) -> (w405:T3)
              n223 = call "CRYAPI SPLITE.vi"("nData"=w410, "sAction"="GET_SPLITER") -> ("tSpliter_Out"=w409:T10)  [unwired: 4 in, 5 out]
              n224 = call "CRYAPI SPLITE.vi"("tSpliter"=w400, "nData"=w399, "sAction"="REMOVE_SPLITER") -> ()  [unwired: 3 in, 6 out]
              n225 = Unbundle By Name(w405) -> ("pSPF"=w404:refnum<vi>)
              n226 = Unbundle By Name(w405) -> ("nID"=w408:i32)
              n227 = Bundle By Name(cluster=w409, "nIDParent"=w408, "nTypeP"=0) -> (w406:T10)
              n228 = invoke class="SubPnl" method="Insert VI"(reference=w404, error in=w403, "VI Ref"=w412) -> (reference out=w419:refnum<vi>, error out=w418:errorcluster)  [unwired: 1 in, 2 out]
              n229 = invoke class="SubPnl" method="FitControlToPane"(reference=w419, error in=w418) -> ()  [unwired: 1 in, 3 out]
              n230 = call "CRYAPI SPLITE.vi"("tSpliter"=w406, "sAction"="REPLACE_SPLITER") -> ()  [unwired: 4 in, 6 out]
              n231 = call "CRYAPI FRAME.vi"("tFrame"=w405, "sAction"="REPLACE_FRAME") -> ()  [unwired: 4 in, 6 out]
            }
            frame "SPLITER" {
              n232 = Unbundle By Name(w435) -> ("nIDParent"=w444:i32)
              n233 = Unbundle By Name(w439) -> ("pSP"=w438:refnum<vi>)
              n234 = call "CRYAPI SPLITE.vi"("nData"=w444, "sAction"="GET_SPLITER") -> ("tSpliter_Out"=w442:T10)  [unwired: 4 in, 5 out]
              n235 = invoke class="SubPnl" method="Remove VI"(reference=w438) -> (reference out=w436:refnum<vi>)  [unwired: 2 in, 2 out]
              n236 = call "CRYAPI SPLITE.vi"("tSpliter_In"=w435, "tSpliter"=w442, "sAction"="GET_SPLITER_LR") -> ("nData_Out"=w437:i32, "tLR_Out"=w440:T12, "tSpliter_Out"=w441:T10)  [unwired: 3 in, 3 out]
              n237 = case shown="0, 1, Default" w437 {
                tunnel: w441 -> [w472 w483]
                tunnel: w440 -> [w470 w481]
                tunnel: [w469 w480] -> w430
                tunnel: w439 -> [w471 w482]
                tunnel: w436 -> [_ _]
                tunnel: w435 -> [w466 w477]
                tunnel: [w468 w479] -> w429
                tunnel: [w467 w478] -> w426
                tunnel: [w466 w477] -> w422
                tunnel: [w463 w474] -> w427
                tunnel: [w462 w473] -> w425
                frame 0, 1, Default {
                  n238 = Unbundle By Name(w470) -> ("pSP"=w469:refnum<vi>)
                  n239 = Unbundle By Name(w471) -> ("pVI"=w468:refnum<vi>, "nIDT"=w465:i32, "nID"=w462:i32)
                  n240 = Equal?(x=w465, y=0) -> (x = y?=w463:bool)
                  n241 = Bundle By Name(cluster=w472, "pVIL"=w468, "nIDTL"=w465, "nIDL"=w462) -> (w467:T10)
                }
                frame 2 {
                  n242 = Unbundle By Name(w481) -> ("pSP"=w480:refnum<vi>)
                  n243 = Unbundle By Name(w482) -> ("pVI"=w479:refnum<vi>, "nIDT"=w476:i32, "nID"=w473:i32)
                  n244 = Equal?(x=w476, y=0) -> (x = y?=w474:bool)
                  n245 = Bundle By Name(cluster=w483, "pVIR"=w479, "nIDTR"=w476, "nIDR"=w473) -> (w478:T10)
                }
              }
              n246 = invoke class="SubPnl" method="Remove VI"(reference=w430) -> (reference out=w434:refnum<vi>, error out=w433:errorcluster)  [unwired: 2 in, 1 out]
              n247 = case shown="False" w427 {
                tunnel: w426 -> [w451 w459]
                tunnel: w425 -> [w452 w460]
                tunnel: [w451 w459] -> w423
                tunnel: w422 -> [w446 w455]
                tunnel: [w446 w455] -> w421
                frame True {
                  n248 = Unbundle By Name(w451) -> ("nID"=w449:i32)
                  n249 = call "CRYAPI FRAME.vi"("nData"=w452, "sAction"="GET_FRAME") -> ("tFrame_Out"=w450:T3)  [unwired: 4 in, 5 out]
                  n250 = Bundle By Name(cluster=w450, "nParent"=w449) -> (w447:T3)
                  n251 = call "CRYAPI FRAME.vi"("tFrame"=w447, "sAction"="REPLACE_FRAME") -> ()  [unwired: 4 in, 6 out]
                }
                frame False {
                  n252 = Unbundle By Name(w459) -> ("nID"=w457:i32)
                  n253 = call "CRYAPI SPLITE.vi"("nData"=w460, "sAction"="GET_SPLITER") -> ("tSpliter_Out"=w458:T10)  [unwired: 4 in, 5 out]
                  n254 = Bundle By Name(cluster=w458, "nIDParent"=w457) -> (w454:T10)
                  n255 = call "CRYAPI SPLITE.vi"("tSpliter"=w454, "sAction"="REPLACE_SPLITER") -> ()  [unwired: 4 in, 6 out]
                }
              }
              n256 = invoke class="SubPnl" method="Insert VI"(reference=w434, error in=w433, "VI Ref"=w429) -> (reference out=w432:refnum<vi>, error out=w431:errorcluster)  [unwired: 1 in, 2 out]
              n257 = invoke class="SubPnl" method="FitControlToPane"(reference=w432, error in=w431) -> ()  [unwired: 1 in, 3 out]
              n258 = call "CRYAPI SPLITE.vi"("tSpliter"=w423, "sAction"="REPLACE_SPLITER") -> ()  [unwired: 4 in, 6 out]
              n259 = call "CRYAPI SPLITE.vi"("tSpliter"=w421, "sAction"="REMOVE_SPLITER") -> ()  [unwired: 4 in, 6 out]
            }
          }
        }
      }
    }
    frame "RECOVERY_FRAMES" {
      n260 = local write "nData_Out"(w484) -> ()
      n261 = call "CRYAPI REMOVE.vi"("sAction"="GET_TAB_FRAMES") -> ("List_ID_Out"=w487:i32[])  [unwired: 4 in, 6 out]
      n262 = call "CRYAPI REMOVE.vi"("sAction"="GET_WIN_FRAMES") -> ("List_ID_Out"=w491:i32[])  [unwired: 4 in, 6 out]
      n263 = call "CRYAPI REMOVE.vi"("sAction"="GET_FRAME_FRAMES") -> ("List_ID_Out"=w486:i32[])  [unwired: 4 in, 6 out]
      n264 = for {
        N -> [w586]
        tunnel: w491 -> [w567] mode=indexing
        tunnel: [w586] -> w490
        n265 = call "CRYAPI FRAME.vi"("nData"=w567, "sAction"="GET_SDATA") -> ("sData_Out"=w568:string)  [unwired: 4 in, 5 out]
        n266 = call "CRYAPI FRAME.vi"("nData"=w567, "sAction"="GET_FRAME") -> ("tFrame_Out"=w571:T3)  [unwired: 4 in, 5 out]
        n267 = Unbundle By Name(w571) -> ("sTemp"=w570:string, "sTitle"=w565:string)
        n268 = call "CRYAPI FRAME.vi"("sData"="WIN_YTITLE", "sAction"="NEW_FRAME") -> ("tFrame_Out"=w585:T3)  [unwired: 4 in, 5 out]
        n269 = call "CRYAPI LOAD.vi"("sTitle"=w565, "sOption"=w568, "sData"=w570, "sAction"="LOAD_VI") -> ("tWindow_Out"=w580:T14)  [unwired: 2 in, 5 out]
        n270 = Unbundle By Name(w585) -> ("pVIW"=w584:refnum<vi>, "pSPW"=w583:refnum<vi>, "pVIF"=w582:refnum<vi>, "pSPF"=w581:refnum<vi>)
        n271 = Unbundle By Name(w580) -> ("sTiltle"=w564:string, "pVI"=w579:refnum<vi>)
        n272 = Bundle By Name(cluster=w571, "sTitle"=w564, "pWVI"=w579, "pVIW"=w584, "pSPW"=w583, "pVIF"=w582, "pSPF"=w581) -> (w573:T3)
        n273 = call "CRYAPI FRAME.vi"("tFrame"=w573, "sAction"="RECOVERY_FRAME") -> ("tFrame_Out"=w574:T3)  [unwired: 4 in, 5 out]
        n274 = call "CRYAPI FRAME.vi"("tFrame"=w574, "sAction"="SET_FRAME" ("string")) -> ("tFrame_Out"=w572:T3)  [unwired: 4 in, 5 out]
        n275 = call "CRYAPI FRAME.vi"("tFrame"=w572, "sAction"="REPLACE_FRAME") -> ("tFrame_Out"=w566:T3)  [unwired: 4 in, 5 out]
        n276 = Unbundle By Name(w566) -> ("pVIW"=w577:refnum<vi>, "Bound"=w562:T1)
        n277 = property class="VI"(reference=w577, "Front Panel.PanelBounds"=w562) -> (error out=w563:errorcluster)  [unwired: 1 in, 1 out]
        n278 = case shown="Error" w563 {
          frame No Error {
          }
          frame Error {
          }
        }
      }
      n279 = for {
        N -> [w561]
        tunnel: [w561] -> w485
        tunnel: w487 -> [w558] mode=indexing
        tunnel: w490 -> [_]
        n280 = call "CRYAPI FRAME.vi"("nData"=w558, "sAction"="GET_FRAME") -> ("tFrame_Out"=w547:T3)  [unwired: 4 in, 5 out]
        n281 = Unbundle By Name(w547) -> ("nType"=w557:i32)
        n282 = Equal To 0?(x=w557) -> (x = 0?=w560:bool)
        n283 = Select(t="TAB_NTITLE" ("sData"), s=w560, f="TAB_YTITLE" ("sData")) -> (s? t:f=w553:string)
        n284 = call "CRYAPI FRAME.vi"("sData"=w553, "sAction"="NEW_FRAME") -> ("tFrame_Out"=w548:T3)  [unwired: 4 in, 5 out]
        n285 = Unbundle By Name(w548) -> ("pVIW"=w552:refnum<vi>, "pSPW"=w551:refnum<vi>, "pVIF"=w550:refnum<vi>, "pSPF"=w549:refnum<vi>, "pTab"=w546:refnum<vi>, "pSPT"=w545:refnum<vi>)
        n286 = Bundle By Name(cluster=w547, "pVIW"=w552, "pSPW"=w551, "pVIF"=w550, "pSPF"=w549, "pTab"=w546, "pSPT"=w545) -> (w541:T3)
        n287 = Unbundle By Name(w541) -> ("pVIF"=w544:refnum<vi>, "nID"=w538:i32)
        n288 = invoke class="VI" method="Ctrl Val.Set"(reference=w544, "Control Name"="WID", "Value"=w538) -> ()  [unwired: 2 in, 5 out]
        n289 = call "CRYAPI FRAME LIB.vi"("tFrame"=w541, "nData"=w538, "sAction"="RECOVERY_PAGES") -> ("tFrame_Out"=w535:T3)  [unwired: 3 in, 5 out]
        n290 = call "CRYAPI FRAME.vi"("tFrame"=w535, "sAction"="SET_FRAME" ("string")) -> ("tFrame_Out"=w534:T3)  [unwired: 4 in, 5 out]
        n291 = Unbundle By Name(w534) -> ("nIDPages"=w530:i32[], "pVIF"=w533:refnum<vi>)
        n292 = call "CRYAPI FRAME.vi"("tFrame"=w534, "sAction"="REPLACE_FRAME") -> ("tFrame_Out"=w540:T3)  [unwired: 4 in, 5 out]
        n293 = Unbundle By Name(w540) -> ("pTab"=w537:refnum<vi>)
        n294 = Sort 1D Array(array=w530) -> (sorted array=w529:i32[])
        n295 = Index Array(array=w529, index=0) -> (element=w527:i32)
        n296 = property class="TabCtl"(reference=w537, "Value"=w527) -> (error out=w526:errorcluster)  [unwired: 1 in, 1 out]
        n297 = invoke class="VI" method="Ctrl Val.Set"(reference=w533, error in=w526, "Control Name"="sMessage", "Value"="REFRESH_PANE" ("sAction")) -> ()  [unwired: 1 in, 5 out]
      }
      n298 = for {
        tunnel: w486 -> [w505] mode=indexing
        tunnel: w485 -> [_]
        n299 = call "CRYAPI FRAME.vi"("nData"=w505, "sAction"="GET_FRAME") -> ("tFrame_Out"=w509:T3)  [unwired: 4 in, 5 out]
        n300 = Unbundle By Name(w509) -> ("sTemp"=w504:string, "nType"=w496:i32, "nID"=w495:i32)
        n301 = case shown="0, Default" w496 {
          tunnel: w495 -> [w519 _]
          tunnel: [w518 "WIN_YTITLE" ("sData")] -> w494
          frame 0, Default {
            n302 = case shown="Default" w519 {
              tunnel: ["WIN_NTITLE" ("sData") "WIN_MTITLE" ("sData")] -> w518
              frame Default {
              }
              frame 1 {
              }
            }
          }
          frame 1, 2 {
          }
        }
        n303 = Not Equal?(x="", y=w504) -> (x != y?=w502:bool)
        n304 = call "CRYAPI FRAME.vi"("sData"=w494, "sAction"="NEW_FRAME") -> ("tFrame_Out"=w508:T3)  [unwired: 4 in, 5 out]
        n305 = case shown="False" w502 {
          tunnel: w504 -> [_ w524]
          tunnel: [_ w523] -> w501
          frame False {
          }
          frame True {
            n306 = call "CRYAPI LOAD.vi"("sData"=w524, "sAction"="LOAD_VI") -> ("tWindow_Out"=w523:T14)  [unwired: 4 in, 5 out]
          }
        }
        n307 = Unbundle By Name(w508) -> ("pVIW"=w510:refnum<vi>, "pSPW"=w511:refnum<vi>, "pVIF"=w512:refnum<vi>, "pSPF"=w513:refnum<vi>)
        n308 = Unbundle By Name(w501) -> ("pVI"=w498:refnum<vi>)
        n309 = Bundle By Name(cluster=w509, "pWVI"=w498, "pVIW"=w510, "pSPW"=w511, "pVIF"=w512, "pSPF"=w513) -> (w499:T3)
        n310 = call "CRYAPI FRAME.vi"("tFrame"=w499, "sAction"="SET_FRAME" ("string")) -> ("tFrame_Out"=w497:T3)  [unwired: 4 in, 5 out]
        n311 = call "CRYAPI FRAME.vi"("tFrame"=w497, "sAction"="REPLACE_FRAME") -> ("tFrame_Out"=w515:T3)  [unwired: 4 in, 5 out]
        n312 = Unbundle By Name(w515) -> ("pVIW"=w516:refnum<vi>, "Bound"=w517:T1)
        n313 = property class="VI"(reference=w516, "Front Panel.PanelBounds"=w517) -> (error out=w493:errorcluster)  [unwired: 1 in, 1 out]
        n314 = case shown="Error" w493 {
          frame No Error {
          }
          frame Error {
          }
        }
      }
    }
    frame "RECOVERY_SPLITERS" {
      n315 = global read "CRYMain Sub Window Global.vi" "cSpliter"() -> (w594:T15)
      n316 = local write "nData_Out"(w591) -> ()
      n317 = global read "CRYMain Sub Window Global.vi" "cSpliter"() -> (w597:T15)
      n318 = Unbundle By Name(w597) -> ("Spliter"=w596:T16)
      n319 = Unbundle By Name(w594) -> ("nID"=w595:i32[])
      n320 = for {
        tunnel: w596 -> [w651] mode=indexing
        tunnel: [w646] -> w593
        tunnel: w592 -> [w644] mode=indexing
        i -> [w646]
        n321 = Unbundle By Name(w644) -> ("Rect"=w643:T1, "nPos"=w642:i32, "Sizing"=w639:T4)
        n322 = Unbundle By Name(w651) -> ("nType"=w645:i32)
        n323 = case shown="0, Default" w645 {
          tunnel: ["NSPLITER" ("sAction") "VSPLITER" ("sAction") "HSPLITER" ("sAction")] -> w653
          frame 0, Default {
          }
          frame 1 {
          }
          frame 2 {
          }
        }
        n324 = call "CRYAPI SPLITE.vi"("sData"=w653, "sAction"="NEW_SPLITER") -> ("tSpliter_Out"=w652:T10)  [unwired: 4 in, 5 out]
        n325 = Unbundle By Name(w652) -> ("pVI"=w641:refnum<vi>, "pSpliter"=w640:refnum<vi>, "pSPL"=w648:refnum<vi>, "pSPR"=w647:refnum<vi>)
        n326 = case shown="1, 2" w645 {
          tunnel: w643 -> [w661 _]
          tunnel: w642 -> [w658 _]
          tunnel: w641 -> [w662 _]
          tunnel: w640 -> [w659 _]
          tunnel: w639 -> [w657 _]
          frame 1, 2 {
            n327 = property class="VI"(reference=w662, "Front Panel.PanelBounds"=w661) -> (error out=w656:errorcluster)  [unwired: 1 in, 1 out]
            n328 = property class="Splitter"(reference=w659, error in=w656, "Position"=w658) -> (reference out=w660:refnum<vi>, error out=w655:errorcluster)
            n329 = case shown="No Error" w655 {
              tunnel: w660 -> [w664 _]
              tunnel: w657 -> [w663 _]
              frame No Error {
                n330 = property class="Splitter"(reference=w664, "Sizing"=w663) -> ()  [unwired: 1 in, 2 out]
              }
              frame Error {
              }
            }
          }
          frame 0, Default {
          }
        }
        n331 = Bundle By Name(cluster=w651, "pVI"=w641, "pSpliter"=w640, "pSPL"=w648, "pSPR"=w647) -> (w649:T10)
        n332 = call "CRYAPI SPLITE.vi"("tSpliter"=w649, "sAction"="REPLACE_SPLITER") -> ()  [unwired: 4 in, 6 out]
      }
      n333 = for {
        tunnel: w595 -> [w599] mode=indexing
        tunnel: w593 -> [_]
        n334 = call "CRYAPI SPLITE.vi"("nData"=w599, "sAction"="GET_SPLITER") -> ("tSpliter_Out"=w598:T10)  [unwired: 4 in, 5 out]
        n335 = Unbundle By Name(w598) -> ("pSPL"=w604:refnum<vi>, "pSPR"=w603:refnum<vi>, "nIDTL"=w612:i32, "nIDL"=w614:i32, "nIDTR"=w611:i32, "nIDR"=w610:i32, "nType"=w605:i32)  [unwired: 1 out]
        n336 = Equal To 0?(x=w612) -> (x = 0?=w613:bool)
        n337 = case shown="1, 2" w605 {
          tunnel: w611 -> [_ w621]
          tunnel: w610 -> [_ w620]
          tunnel: [refnum<vi> refnum ("pVIW") w619] -> w609
          tunnel: w603 -> [_ w618]
          frame 0, Default {
          }
          frame 1, 2 {
            n338 = Equal To 0?(x=w621) -> (x = 0?=w622:bool)
            n339 = case shown="False" w622 {
              tunnel: w620 -> [w625 w629]
              tunnel: [w623 w627] -> w619
              frame False {
                n340 = call "CRYAPI SPLITE.vi"("nData"=w625, "sAction"="GET_SPLITER") -> ("tSpliter_Out"=w624:T10)  [unwired: 4 in, 5 out]
                n341 = Unbundle By Name(w624) -> ("pVI"=w623:refnum<vi>)
              }
              frame True {
                n342 = call "CRYAPI FRAME.vi"("nData"=w629, "sAction"="GET_FRAME") -> ("tFrame_Out"=w628:T3)  [unwired: 4 in, 5 out]
                n343 = Unbundle By Name(w628) -> ("pVIW"=w627:refnum<vi>)
              }
            }
            n344 = invoke class="SubPnl" method="Insert VI"(reference=w618, "VI Ref"=w619) -> (reference out=w617:refnum<vi>, error out=w616:errorcluster)  [unwired: 2 in, 2 out]
            n345 = invoke class="SubPnl" method="FitControlToPane"(reference=w617, error in=w616) -> ()  [unwired: 1 in, 3 out]
          }
        }
        n346 = case shown="True" w613 {
          tunnel: w614 -> [w633 w637]
          tunnel: [w631 w635] -> w606
          frame False {
            n347 = call "CRYAPI SPLITE.vi"("nData"=w633, "sAction"="GET_SPLITER") -> ("tSpliter_Out"=w632:T10)  [unwired: 4 in, 5 out]
            n348 = Unbundle By Name(w632) -> ("pVI"=w631:refnum<vi>)
          }
          frame True {
            n349 = call "CRYAPI FRAME.vi"("nData"=w637, "sAction"="GET_FRAME") -> ("tFrame_Out"=w636:T3)  [unwired: 4 in, 5 out]
            n350 = Unbundle By Name(w636) -> ("pVIW"=w635:refnum<vi>)
          }
        }
        n351 = invoke class="SubPnl" method="Insert VI"(reference=w604, "VI Ref"=w606) -> (reference out=w602:refnum<vi>, error out=w601:errorcluster)  [unwired: 2 in, 2 out]
        n352 = Bundle By Name(cluster=w598, "pVIL"=w606, "pVIR"=w609) -> (w607:T10)
        n353 = invoke class="SubPnl" method="FitControlToPane"(reference=w602, error in=w601) -> ()  [unwired: 1 in, 3 out]
        n354 = call "CRYAPI SPLITE.vi"("tSpliter"=w607, "sAction"="REPLACE_SPLITER") -> ()  [unwired: 4 in, 6 out]
      }
    }
    frame "RESPLITE_FRAME" {
      n355 = call "CRYAPI FRAME.vi"("nData"=w673, "sAction"="GET_FRAME") -> ("tFrame_Out"=w671:T3)  [unwired: 4 in, 5 out]
      n356 = call "CRYAPI REMOVE.vi"("tFrame"=w671, "sAction"="GET_LIST_ID") -> ("List_ID_Out"=w669:i32[])  [unwired: 3 in, 6 out]
      n357 = call "CRYAPI REMOVE.vi"("List_ID"=w669, "sAction"="GET_LIST_IDSPLITER") -> ("List_ID_Out"=w668:i32[])  [unwired: 3 in, 6 out]
      n358 = for {
        tunnel: w668 -> [w684] mode=indexing
        n359 = call "CRYAPI SPLITE.vi"("nData"=w684, "sAction"="GET_SPLITER") -> ("tSpliter_Out"=w687:T10)  [unwired: 4 in, 5 out]
        n360 = Unbundle By Name(w687) -> ("pSpliter"=w680:refnum<vi>, "nType"=w685:i32, "pVI"=w686:refnum<vi>)  [unwired: 2 out]
        n361 = case shown="1, Default" w685 {
          tunnel: w686 -> [w698 w706]
          tunnel: [w692 w700] -> w683
          tunnel: [w691 w699] -> w677
          tunnel: w680 -> [w691 w699]
          frame 1, Default {
            n362 = property class="VI"(reference=w698) -> ("Front Panel.PanelBounds"=w697:T1)  [unwired: 1 in, 2 out]
            n363 = Unbundle By Name(w697) -> ("Right"=w695:i16, "Left"=w696:i16, "Bottom"=w694:i16, "Top"=w693:i16)
            n364 = Subtract(x=w695, y=w696) -> (x-y=w692:i16)
            n365 = Subtract(x=w694, y=w693) -> ()  [unwired: 1 out]
          }
          frame 2 {
            n366 = property class="VI"(reference=w706) -> ("Front Panel.PanelBounds"=w705:T1)  [unwired: 1 in, 2 out]
            n367 = Unbundle By Name(w705) -> ("Right"=w703:i16, "Left"=w704:i16, "Bottom"=w702:i16, "Top"=w701:i16)
            n368 = Subtract(x=w703, y=w704) -> ()  [unwired: 1 out]
            n369 = Subtract(x=w702, y=w701) -> (x-y=w700:i16)
          }
        }
        n370 = Divide(x=w683, y=i16 2) -> (x/y=w681:dbl)
        n371 = To Long Integer(number=w681) -> (32bit integer=w679:i32)
        n372 = property class="Splitter"(reference=w677, "Position"=w679) -> (reference out=w678:refnum<vi>, error out=w675:errorcluster)  [unwired: 1 in]
        n373 = property class="Splitter"(reference=w677) -> ("Sizing"=w676:T4)  [unwired: 1 in, 2 out]
        n374 = case shown="No Error" w675 {
          tunnel: w678 -> [w690 _]
          tunnel: w676 -> [w689 _]
          frame No Error {
            n375 = property class="Splitter"(reference=w690, "Sizing"=w689) -> ()  [unwired: 1 in, 2 out]
          }
          frame Error {
          }
        }
      }
    }
    frame "FIND_TOP_VI" {
      n376 = global read "CRYMain Sub Window Global.vi" "cFrame"() -> (w712:T8)
      n377 = Unbundle By Name(w712) -> ("Frame"=w711:T9)
      n378 = for {
        tunnel: w711 -> [w722] mode=indexing
        shift-right: [w716] -> w707
        shift-left: -1 -> [w717]
        shift-right: [w713] -> w708
        shift-left: T3 {"nType"=0, "nParent"=0, "pVIW"=refnum, "pSPW"=refnum, "nTypeF"=0, "pVIF"=refnum, "pSPF"=refnum, "nIDSpliter"=0, "nProperty"=0, "Bound"={"Left"=0, "Top"=0, "Right"=0, "Bottom"=0}, "nID"=0, "nData"=0, "sData"="", "pWVI"=refnum, "sTitle"="", "cPages"=[], "pTab"=refnum, "nIDPages"=[], "pSPT"=refnum, "sTemp"="", "nDockID"=0, "nDockLR"=0, "sIcon"=""} ("tFrame_Out") -> [w714]
        n379 = Unbundle By Name(w722) -> ("nType"=w721:i32, "nParent"=w723:i32, "nID"=w715:i32)
        n380 = Equal To 0?(x=w723) -> (x = 0?=w719:bool)
        n381 = Not Equal To 0?(x=w721) -> (x != 0?=w720:bool)
        n382 = And(x=w720, y=w719) -> (x .and. y?=w718:bool)
        n383 = case shown="True" w718 {
          tunnel: w722 -> [_ w726]
          tunnel: w717 -> [w725 w731]
          tunnel: [w725 w729] -> w716
          tunnel: w715 -> [_ _]
          tunnel: w714 -> [w724 w728]
          tunnel: [w724 w727] -> w713
          frame False {
          }
          frame True {
            n384 = Unbundle By Name(w726) -> ("pVIW"=w736:refnum<vi>)
            n385 = invoke class="VI" method="Ctrl Val.Get"(reference=w736, "Control Name"="ActiveNumber") -> ("Get Control Value Variant"=w734:variant)  [unwired: 2 in, 3 out]
            n386 = Variant To Data(type=0, Variant=w734) -> (data=w730:i32)  [unwired: 1 in, 1 out]
            n387 = Greater?(x=w730, y=w731) -> (0:w732:bool)
            n388 = case shown="True" w732 {
              tunnel: w731 -> [w738 _]
              tunnel: w730 -> [_ w740]
              tunnel: [w738 w740] -> w729
              tunnel: w728 -> [w737 _]
              tunnel: [w737 w739] -> w727
              tunnel: w726 -> [_ w739]
              frame False {
              }
              frame True {
              }
            }
          }
        }
      }
      n389 = local write "tFrame_Out"(w708) -> ()
      n390 = local write "nData_Out"(w707) -> ()
    }
  }
